vi "ReadBuffer.vi"(8 "Uart Input":cluster{u64}={365647016} {"?" format="%x"}, 10 "Buffer Size":u32=64, 11 "Error Input":errorcluster) -> (0 "Uart Output":cluster{u64}={365647016} {"?" format="%x"}, 1 "String Buffer":string, 2 "Byte Buffer":u8[](array[numeric])=[69, 67, 67, 45, 76, 97, 98, 46, 13, 10, 0, 0, 0, 0, 0, 0, 0, 0, 0, 0, 0, 0, 0, 0, 0, 0, 0, 0, 0, 0, 0, 0, 0, 0, 0, 0, 0, 0, 0, 0, 0, 0, 0, 0, 0, 0, 0, 0, 0, 0, 0, 0, 0, 0, 0, 0, 0, 0, 0, 0, 0, 0, 0, 0] format="%x", 3 "Error Output":errorcluster, 4 "Line String":string)   [LabVIEW 2019]
doc: "<B>Read</B> internal bytes buffer of the serial port. The internal bytes buffer will be cleared automatically."
uses:
  dll/LabViewUart.dll
panel:
  # "Read Bytes Buffer"
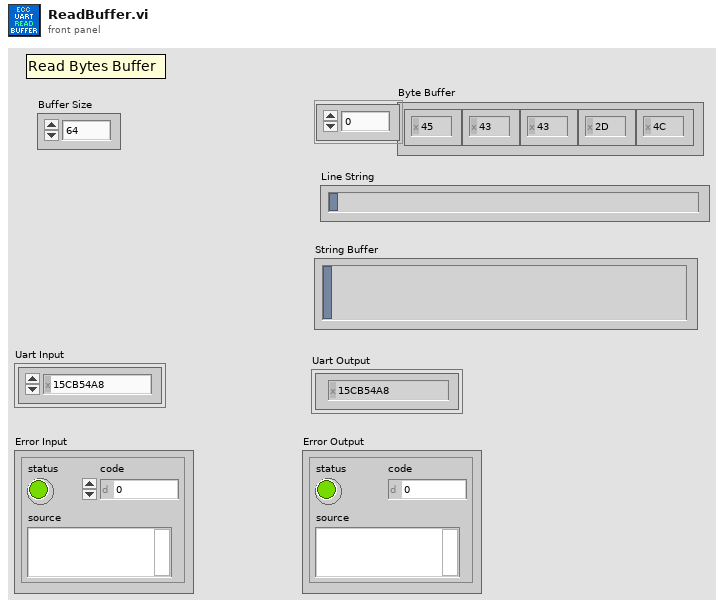
[diagram p1: front panel]
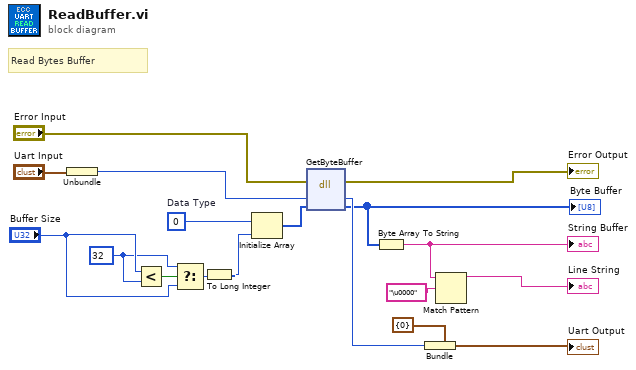
[diagram p0: block diagram]
diagram:
  w17 = u32 32 ("y")
  w14 = u8 0  # Data Type
  # "Read Bytes Buffer"
  n1 = Unbundle("Uart Input") -> (w11:u64)
  n2 = Less?(x="Buffer Size", y=w17) -> (x < y?=w16:bool)
  n3 = Select(t=w17, s=w16, f="Buffer Size") -> (s? t:f=w6:u32)
  n4 = To Long Integer(number=w6) -> (32bit integer=w5:i32)
  n5 = Initialize Array(w14, w5) -> (w15:u8[])
  n6 = dll-call lib="D:/Google Drive/INC-2020/INC352/INC352-2020/LabVIEW/examples/uart-cmdex/SubVI/dll/LabViewUart.dll" fn="GetByteBuffer"(error in="Error Input", "Object Handle"=w11, "Byte Buffer"=w15) -> (error out=→"Error Output":errorcluster, "Object Handle"=w9:u64, "Byte Buffer"=w4:u8[])  [unwired: 3 in, 1 out]
  "Byte Buffer" <- w4
  n7 = Byte Array To String(unsigned byte array=w4) -> (string=w1:string)
  "String Buffer" <- w1
  n8 = Bundle(cluster=cluster{u64} {0}, w9) -> (→"Uart Output":cluster{u64})
  n9 = Match Pattern(string=w1, regular expression="\u0000") -> (before substring=→"Line String":string)  [unwired: 1 in, 3 out]
